vi "email notification.vi"   [LabVIEW 2016]
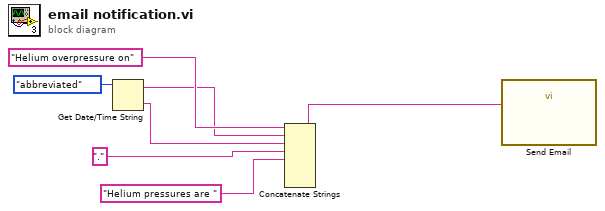
[diagram p0: block diagram]
diagram:
  n1 = Get Date/Time String(date format (0)=enum16{"short", "long", "abbreviated"}."abbreviated") -> (date string=w4:string, time string=w3:string)  [unwired: 2 in]
  n2 = Concatenate Strings("Helium overpressure on", w4, w3, "." ("string"), "Helium pressures are " ("string")) -> (w6:string)  [unwired: 3 in]
  n3 = call "Send Email"("Message"=w6) -> ()  [unwired: 10 in, 1 out]
